vi "Exit.vi"(8 "error in (no error)":errorcluster, 11 "Data":variant) -> (0 "error out":errorcluster)   [LabVIEW 2020, in "Control.lvlib"]
doc: "For named purposes"
uses:
  Control.lvlib
  Private Control/Queue Element.ctl
  Private Control/Module Action.ctl
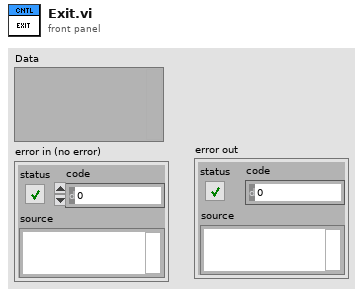
[diagram p1: front panel]
types:
  T1 = typedef "Control.lvlib/Queue Element.ctl" = cluster{"Module Action":T2, "Data":variant}
  T2 = typedef "Control.lvlib/Module Action.ctl" = enum16{"Init", "Termination ", "Error", "Exit"}
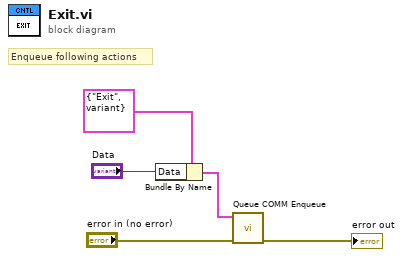
[diagram p0: block diagram]
diagram:
  # "Enqueue following actions"
  n1 = Bundle By Name(cluster=T1 {"Module Action"=enum."Exit", "Data"=variant} ("element"), "Data"="Data") -> (w3:T1)
  n2 = call "Queue COMM Enqueue.vi"("error in (no error)"="error in (no error)", "element"=w3) -> ("error out"=→"error out":errorcluster)  [unwired: 9 in]
